vi "test Modify Alias and Pin.vi"(8 "error in (no error)":errorcluster, 11 "TestCase in":refnum<class "Switch Scripting Unit Tests.lvclass">) -> (0 "error out":errorcluster, 3 "TestCase out":refnum<class "Switch Scripting Unit Tests.lvclass">)   [LabVIEW 2017, in "Switch Scripting Unit Tests.lvclass"]
uses:
  Switch Scripting Unit Tests.lvclass
  Switch Scripting Unit Tests.lvclass/Switch Scripting Unit Tests.ctl
  <vilib>/addons/_JKI Toolkits/VI Tester/TestCase.llb/TestCase.lvclass
  Switch Scripting.lvlib
  C:/Program Files (x86)/National Instruments/LabVIEW 2017/vi.lib/addons/_JKI Toolkits/VI Tester/TestCase.llb/TestCase.lvclass
panel:
  in  "Save?":bool
  out "Output Filename":string
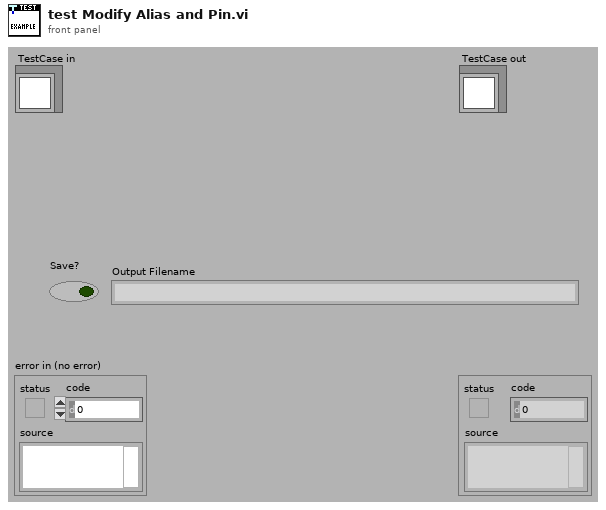
[diagram p1: front panel]
types:
  T1 = typedef "Custom Device API.lvlib/Custom Device Item Ref.ctl" = u64
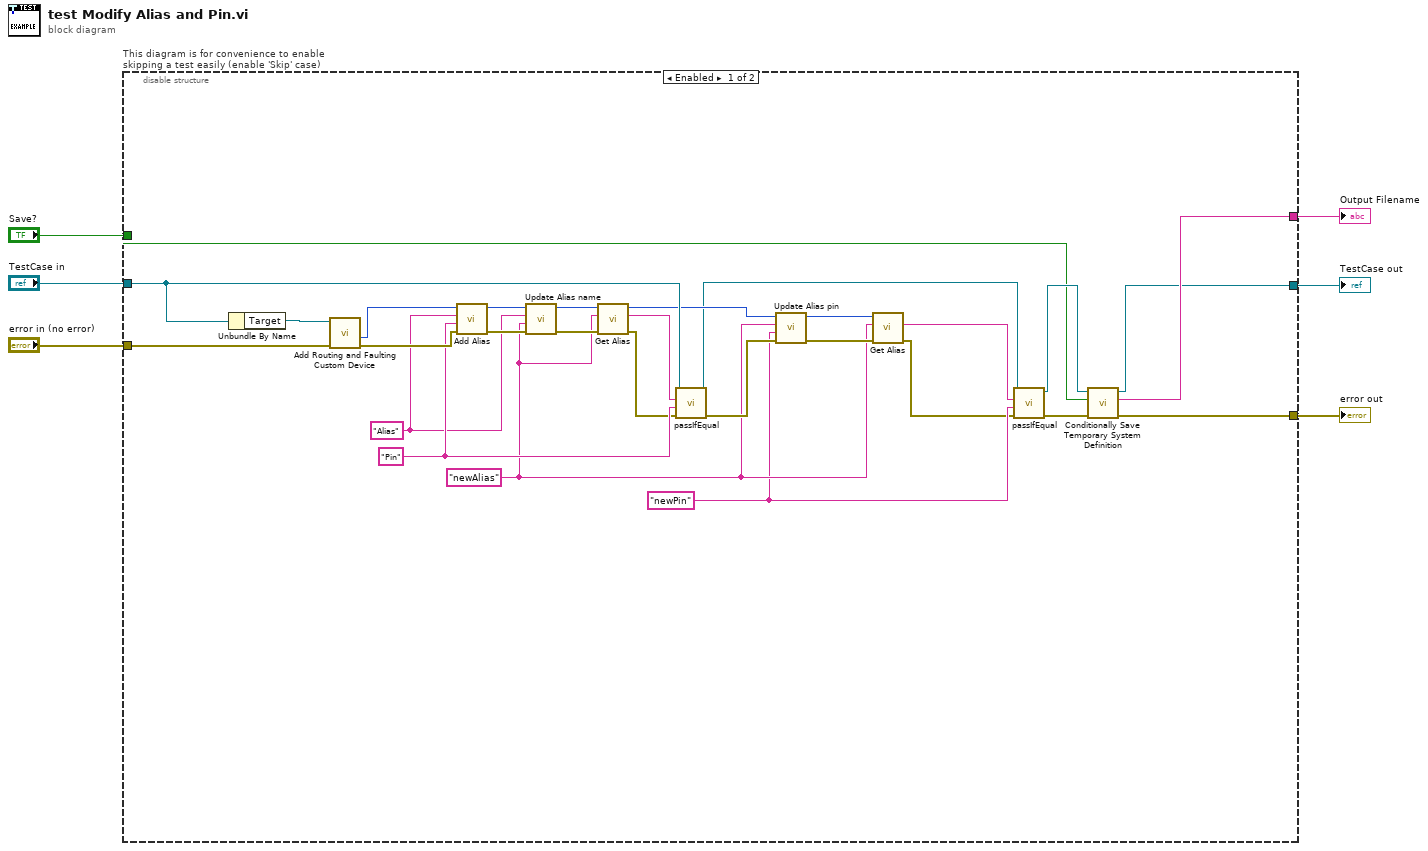
[diagram p0: block diagram]
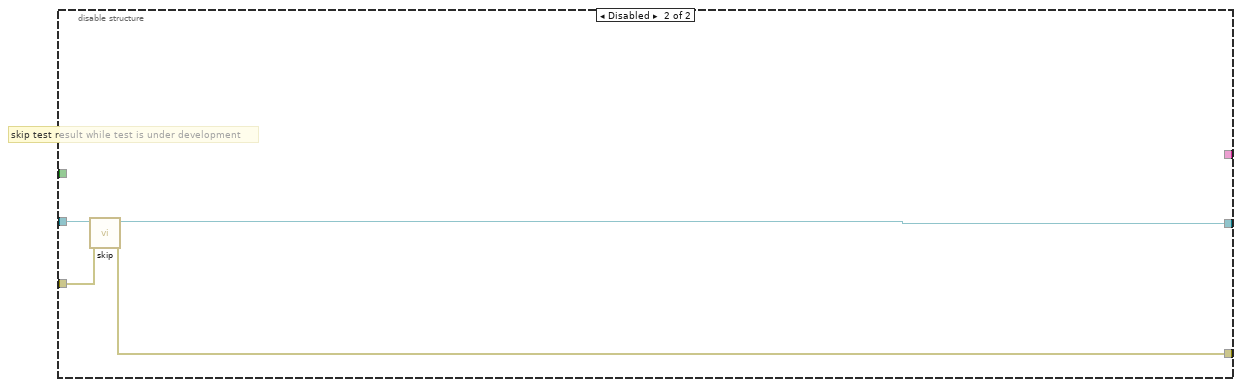
[diagram p2: hidden frame]
diagram:
  n1 = disable-structure "This diagram is for convenience to enable skipping a test easily (enable 'Skip' case)" shown="Enabled" {
    disable-tunnel: "TestCase in" -> [w28 w38]
    disable-tunnel: [w32 w36] -> w3
    disable-tunnel: [w33 w37] -> w5
    disable-tunnel: "error in (no error)" -> [w30 w35]
    disable-tunnel: [w34 _] -> w2
    disable-tunnel: "Save?" -> [w7 _]
    frame Enabled {
      w9 = "newPin" ("Pin")
      w12 = "newAlias" ("Alias")
      w25 = "Pin" ("Pin")
      w17 = "Alias" ("Alias")
      n2 = Unbundle By Name(w28) -> ("Target"=w31:refnum<k24>)
      n3 = call "Add Routing and Faulting Custom Device.vi"("error in (no error)"=w30, "Target in"=w31) -> ("error out"=w27:errorcluster, "Aliases Section Ref"=w29:T1)  [unwired: 5 in, 3 out]
      n4 = call "Add Alias.vi"("error in (no error)"=w27, "Pin"=w25, "Alias"=w17, "Aliases Ref in"=w29) -> ("error out"=w19:errorcluster, "Aliases Ref out"=w21:T1)  [unwired: 6 in]
      n5 = call "Update Alias name.vi"("error in (no error)"=w19, "New Alias name"=w12, "Alias"=w17, "Aliases Ref in"=w21) -> ("error out"=w18:errorcluster, "Aliases Ref out"=w20:T1)  [unwired: 6 in]
      n6 = call "Get Alias.vi"("error in (no error)"=w18, "Alias"=w12, "Aliases Ref in"=w20) -> ("error out"=w24:errorcluster, "Pin"=w26:string, "Aliases Ref out"=w16:T1)  [unwired: 5 in, 1 out]
      n7 = call-dynamic "passIfEqual.vi"("error in (no error)"=w24, "y"=w25, "x"=w26, "TestCase in"=w28) -> ("error out"=w15:errorcluster, "TestCase out"=w11:refnum<class "Switch Scripting Unit Tests.lvclass">)  [unwired: 6 in]
      n8 = call "Update Alias pin.vi"("error in (no error)"=w15, "New Pin"=w9, "Alias"=w12, "Aliases Ref in"=w16) -> ("error out"=w13:errorcluster, "Aliases Ref out"=w14:T1)  [unwired: 5 in, 1 out]
      n9 = call "Get Alias.vi"("error in (no error)"=w13, "Alias"=w12, "Aliases Ref in"=w14) -> ("error out"=w8:errorcluster, "Pin"=w10:string)  [unwired: 5 in, 2 out]
      n10 = call-dynamic "passIfEqual.vi"("error in (no error)"=w8, "y"=w9, "x"=w10, "TestCase in"=w11) -> ("error out"=w22:errorcluster, "TestCase out"=w23:refnum<class "Switch Scripting Unit Tests.lvclass">)  [unwired: 6 in]
      n11 = call "Conditionally Save Temporary System Definition.vi"("error in (no error)"=w22, "Save?"=w7, "Test Case"=w23) -> ("error out"=w33:errorcluster, "filename"=w34:string, "Test Case"=w32:refnum<class "Switch Scripting Unit Tests.lvclass">)  [unwired: 6 in]
    }
    frame Disabled {
      # "skip test result while test is under development"
      n12 = call <vilib>:"skip.vi"("error in (no error)"=w35, "TestCase in"=w38) -> ("error out"=w37:errorcluster, "TestCase out"=w36:refnum<class "Switch Scripting Unit Tests.lvclass">)  [unwired: 8 in]
    }
  }
  "error out" <- w5
  "TestCase out" <- w3
  "Output Filename" <- w2
